vi "Write.vi"(8 "Error In":errorcluster, 10 "Data":u8[](array[numeric]), 11 "SFTP File In":refnum<class "SFTP File.lvclass">) -> (0 "Error Out":errorcluster, 2 "Count":i64, 3 "SFTP File Out":refnum<class "SFTP File.lvclass">)   [LabVIEW 2021, in "Field_RnD_Services_LIBSSH2_Toolkit.lvlib" / "SFTP File.lvclass"]
doc: "Writes a libssh2-defined maximum of 30KB to a remote SFTP file. If more the data is greater than 30kB, then the <B>Write All</B> VI should be used."
uses:
  SFTP File.lvclass
  SFTP File.lvclass/SFTP File.ctl
  Field_RnD_Services_LIBSSH2_Toolkit.lvlib
  SFTP/SFTP.lvclass
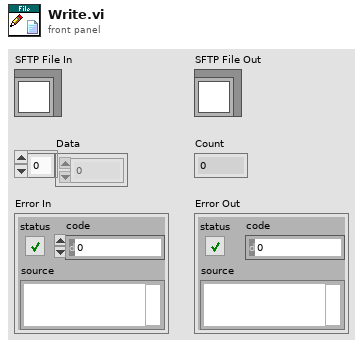
[diagram p1: front panel]
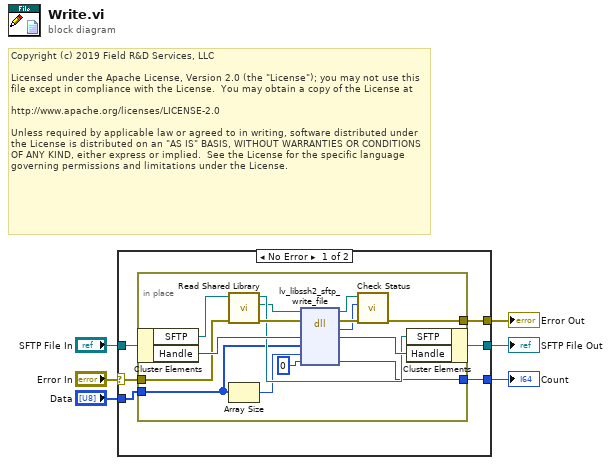
[diagram p0: block diagram]
diagram:
  # "Copyright (c) 2019 Field R&D Services, LLC\n\nLicensed under the Apache License, Version 2.0 (the \"License\"); you may not use this file except in compliance with the License.  You may obtain a copy of the License at\n\nhttp://www.apache.org/licenses/LICENSE-2.0\n\nUnless required by applicable law or agreed to in writing, software distributed under the License is distributed on an \"AS IS\" BASIS, WITHOUT WARRANTIES OR CONDITIONS OF ANY KIND, either express or implied.  See the License for the specific language governing permissions and limitations under the License."
  n1 = case shown="No Error" "Error In" {
    selector: "Error In" -> [w11 w28]
    tunnel: "SFTP File In" -> [w12 w29]
    tunnel: [w10 w29] -> w3
    tunnel: [w9 w28] -> w4
    tunnel: "Data" -> [w8 _]
    tunnel: [w7 _] -> w1
    frame No Error {
      n2 = in-place {
        in-place-border: w11 -> [w26]
        in-place-border: [w21] -> w9
        in-place-border: w8 -> [w15]
        in-place-border: [w13] -> w7
        n3 = in-place-cluster #1(w12) -> ("SFTP"=w18:refnum<class "SFTP.lvclass">, "Handle"=w27:u64)
        n4 = call "Read Shared Library.vi"("Error In"=w26, "SFTP In"=w18) -> ("Erorr Out"=w19:errorcluster, "libssh2lv Shared Library"=w16:path, "SFTP Out"=w17:refnum<class "SFTP.lvclass">)  [unwired: 7 in]
        n5 = Array Size(array=w15) -> (size(s)=w14:i32)
        n6 = dll-call lib="libssh2lv.*" fn="lv_libssh2_sftp_write_file"(path in=w16, error in=w19, "handle"=w27, "buffer"=w15, "buffer_length"=w14, "write_count"=i64 0 ("read_count")) -> (path out=w23:path, error out=w24:errorcluster, "status"=w22:i32, "handle"=w25:u64, "write_count"=w13:i64)  [unwired: 3 in]
        n7 = call "Check Status.vi"("Error In"=w24, "Status"=w22, "libssh2lv Shared Library In"=w23) -> ("Error Out"=w21:errorcluster)  [unwired: 7 in, 1 out]
        n8 = in-place-cluster #1("SFTP"=w17, "Handle"=w25) -> (w10:refnum<class "SFTP File.lvclass">)
      }
    }
    frame Error {
    }
  }
  "Error Out" <- w4
  "SFTP File Out" <- w3
  "Count" <- w1
